vi "parse_details_from_image_name.vi"(8 "Error In":errorcluster, 11 "Image Name":string) -> (0 "Error Out":errorcluster, 3 "Image Properties":T1)   [LabVIEW 2019]
uses:
  git_repos/CAxis_Machine/C-Axis Analysis Program/image_property_cluster_typedef.ctl
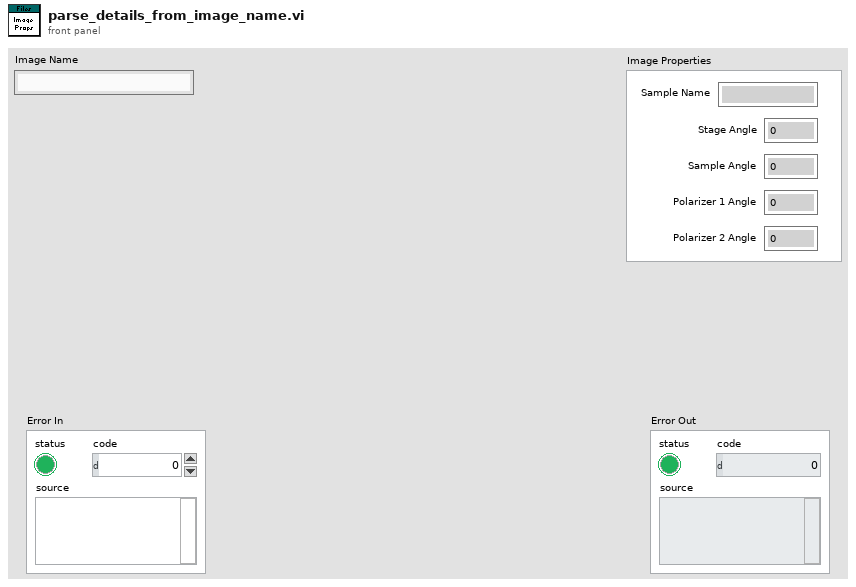
[diagram p1: front panel]
types:
  T1 = typedef "image_property_cluster_typedef.ctl" = cluster{"Stage Angle":dbl, "Sample Angle":dbl, "Polarizer 1 Angle":dbl, "Polarizer 2 Angle":dbl, "Sample Name":string}
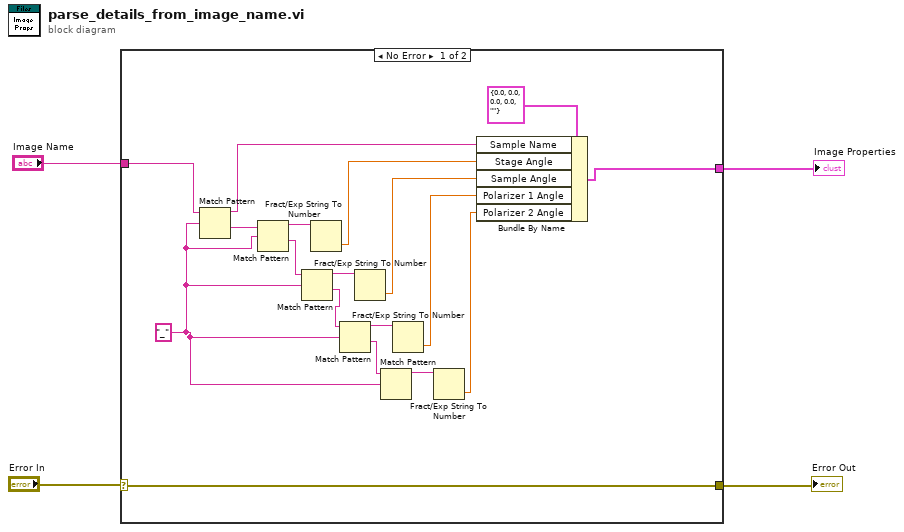
[diagram p0: block diagram]
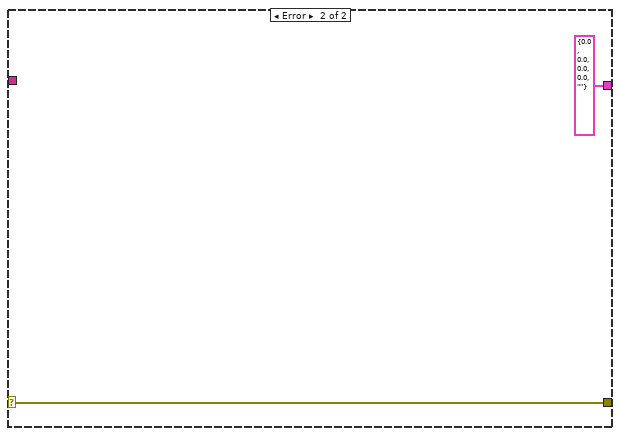
[diagram p2: hidden frame]
diagram:
  n1 = case shown="No Error" "Error In" {
    selector: "Error In" -> [w15 w24]
    tunnel: [w15 w24] -> w3
    tunnel: "Image Name" -> [w22 _]
    tunnel: [w16 T1 {"Stage Angle"=0.0, "Sample Angle"=0.0, "Polarizer 1 Angle"=0.0, "Polarizer 2 Angle"=0.0, "Sample Name"=""} ("Image Properties")] -> w1
    frame No Error {
      w11 = "_" ("regular expression")
      n2 = Match Pattern(string=w22, regular expression=w11) -> (before substring=w20:string, after substring=w19:string)  [unwired: 1 in, 2 out]
      n3 = Match Pattern(string=w19, regular expression=w11) -> (before substring=w18:string, after substring=w14:string)  [unwired: 1 in, 2 out]
      n4 = Match Pattern(string=w14, regular expression=w11) -> (before substring=w13:string, after substring=w10:string)  [unwired: 1 in, 2 out]
      n5 = Fract/Exp String To Number(string=w18) -> (number=w17:dbl)  [unwired: 3 in, 1 out]
      n6 = Match Pattern(string=w10, regular expression=w11) -> (before substring=w8:string, after substring=w9:string)  [unwired: 1 in, 2 out]
      n7 = Fract/Exp String To Number(string=w13) -> (number=w12:dbl)  [unwired: 3 in, 1 out]
      n8 = Match Pattern(string=w9, regular expression=w11) -> (before substring=w7:string)  [unwired: 1 in, 3 out]
      n9 = Fract/Exp String To Number(string=w8) -> (number=w6:dbl)  [unwired: 3 in, 1 out]
      n10 = Fract/Exp String To Number(string=w7) -> (number=w5:dbl)  [unwired: 3 in, 1 out]
      n11 = Bundle By Name(cluster=T1 {"Stage Angle"=0.0, "Sample Angle"=0.0, "Polarizer 1 Angle"=0.0, "Polarizer 2 Angle"=0.0, "Sample Name"=""} ("Image Properties"), "Sample Name"=w20, "Stage Angle"=w17, "Sample Angle"=w12, "Polarizer 1 Angle"=w6, "Polarizer 2 Angle"=w5) -> (w16:T1)
    }
    frame Error {
    }
  }
  "Image Properties" <- w1
  "Error Out" <- w3
